vi "Global Var.vi"() -> ()   [LabVIEW 2016]
panel:
  in  "Waveforms":cluster{waveform(dbl)[]}[](array[cluster])
  in  "Names":string[](array[string])
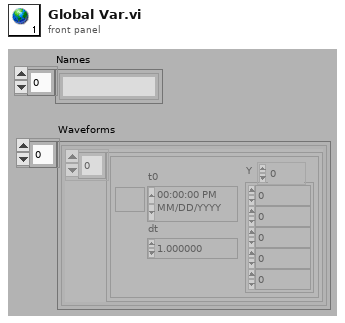
[diagram p1: front panel]
diagram:
